vi "ep_Compute Third Current.vi"   [LabVIEW 2011, in "NI_EP_Power Quality.lvlib"]
uses:
  <vilib>/addons/Electrical Power/PQ/NI_EP_Power Quality.lvlib
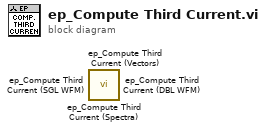
[diagram p0: block diagram]
diagram:
  n1 = call <vilib>:"ep_Compute Third Current (Spectra).vi"() -> ()  [unwired: 14 in, 2 out]
  n2 = call <vilib>:"ep_Compute Third Current (Vectors).vi"() -> ()  [unwired: 14 in, 2 out]
  n3 = call <vilib>:"ep_Compute Third Current (SGL WFM).vi"() -> ()  [unwired: 14 in, 2 out]
  n4 = call <vilib>:"ep_Compute Third Current (DBL WFM).vi"() -> ()  [unwired: 14 in, 2 out]
